vi "svl_Limit Testing with Checks (array) (scalar limits).vi"(0 "upper limit":dbl format="%.2f", 5 "input array":dbl[](array[numeric]) format="%.2f", 7 "lower limit":dbl format="%.2f", 11 "error in (no error)":errorcluster) -> (4 "upper limit array":dbl[](array[numeric]) format="%.2f", 6 "failure array":dbl[](array[numeric]) format="%.2f", 8 "lower limit array":dbl[](array[numeric]) format="%.2f", 13 "test results":bool[](array[boolean]), 14 "test passed":bool, 15 "error out":errorcluster)   [LabVIEW 2017, in "SoundVib_LimitTest.lvlib"]
uses:
  <vilib>/addons/Sound and Vibration/svt_Limit Test/SoundVib_LimitTest.lvlib
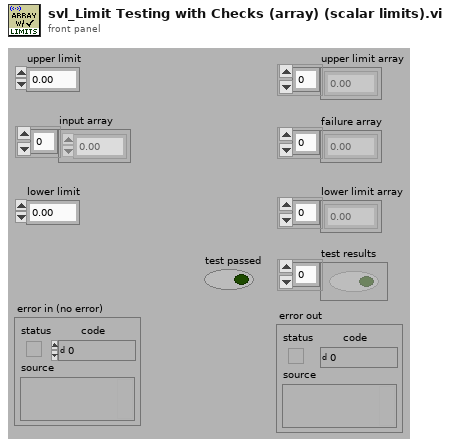
[diagram p1: front panel]
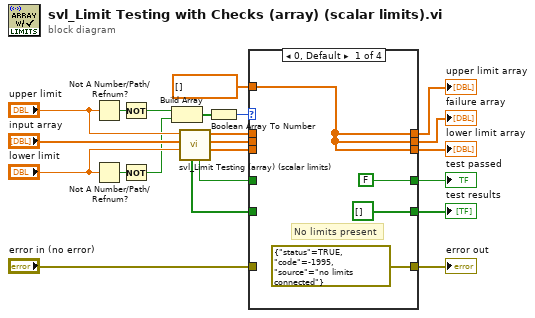
[diagram p0: block diagram]
diagram:
  n1 = Not A Number/Path/Refnum?(number/path/refnum="upper limit") -> (NaN/Path/Refnum?=w8:bool)
  n2 = Not A Number/Path/Refnum?(number/path/refnum="lower limit") -> (NaN/Path/Refnum?=w10:bool)
  n3 = Not(x=w8) -> (.not. x?=w9:bool)
  n4 = Not(x=w10) -> (.not. x?=w11:bool)
  n5 = Build Array(w9, w11) -> (w7:bool[])
  n6 = call <vilib>:"svl_Limit Testing (array) (scalar limits).vi"("lower limit"="lower limit", "input array"="input array", "upper limit"="upper limit") -> ("lower limit array"=w18:dbl[], "failure array"=w17:dbl[], "upper limit array"=w16:dbl[], "test passed"=w19:bool, "test results"=w20:bool[])  [unwired: 4 in]
  n7 = Boolean Array To Number(Boolean array=w7) -> (number=w6:u32)
  n8 = case shown="0, Default" w6 {
    tunnel: w17 -> [_ w29 w36 w43]
    tunnel: [bool[] [] ("test results") w30 w34 w39] -> w12
    tunnel: "error in (no error)" -> [_ w32 w38 w44]
    tunnel: [errorcluster {"status"=TRUE, "code"=-1995, "source"="no limits connected"} ("error IO") w32 w38 w44] -> w2
    tunnel: [FALSE ("test passed") w31 w35 w40] -> w13
    tunnel: w16 -> [_ w28 _ w42]
    tunnel: w18 -> [_ _ w37 w41]
    tunnel: w19 -> [_ w31 w35 w40]
    tunnel: w20 -> [_ w30 w34 w39]
    tunnel: dbl[] [] ("spectrum") -> [w25 w27 w33 _]
    tunnel: [w25 w28 w33 w42] -> w5
    tunnel: [w25 w29 w36 w43] -> w4
    tunnel: [w25 w27 w37 w41] -> w3
    frame 0, Default {
      # "No limits present"
    }
    frame 1 {
      # "Upper limit present\nlower limit absent"
    }
    frame 2 {
      # "Lower limit present\nupper limit absent"
    }
    frame 3 {
      # "upper and lower limits present"
    }
  }
  "failure array" <- w4
  "lower limit array" <- w3
  "upper limit array" <- w5
  "test passed" <- w13
  "test results" <- w12
  "error out" <- w2
